vi "插入数据库.vi"(8 "时间戳":string, 9 "插入数值":string[](array[string]), 10 "table":string="多参数", 11 "database":string="database1.mdb") -> ()   [LabVIEW 2016]
uses:
  <vilib>/Utility/sysdir.llb/System Directory Type.ctl
  <vilib>/addons/database/Connection.llb/DB Tools Open Connec (String).vi
  <vilib>/addons/database/Connection.llb/Conn Execute.vi
  <vilib>/addons/database/Recordset.llb/Rec Destroy - Connection.vi
  <vilib>/addons/database/NI_Database_API.lvlib
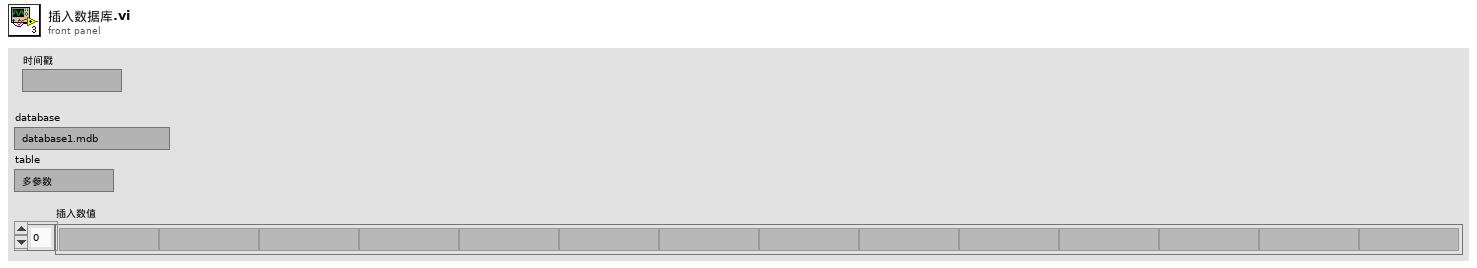
[diagram p1: front panel]
types:
  T1 = typedef "System Directory Type.ctl" = i32
  T2 = typedef "NI_Database_API.lvlib/Conn ObjectReference.ctl" = refnum<k1>
  T3 = typedef "NI_Database_API.lvlib/Rec ObjectReference.ctl" = refnum<k1>
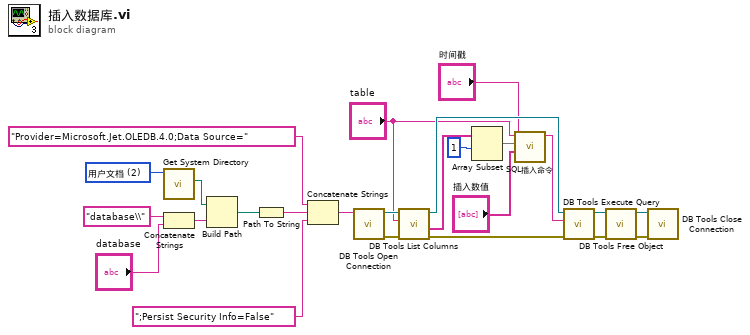
[diagram p0: block diagram]
diagram:
  w21 = T1 2 items=["用户目录"=0, "用户桌面"=1, "用户文档"=2, "用户应用程序数据"=3, "用户设置"=4, "用户临时目录"=5, "公共文档"=6, "公共应用程序数据"=7, "公共设置"=8, "公共缓存"=13, "系统核心库"=9, "系统安装库"=10, "应用程序文件"=11, "启动盘根目录"=12] ("system directory type")
  n1 = call <vilib>:"Get System Directory.vi"("system directory type"=w21) -> ("system directory"=w20:path)  [unwired: 10 in]
  n2 = Concatenate Strings("database\\" ("名称或相对路径"), "database") -> (w4:string)
  n3 = Build Path(base path=w20, name or relative path=w4) -> (appended path=w22:path)
  n4 = Path To String(path=w22) -> (string=w23:string)
  n5 = Concatenate Strings("Provider=Microsoft.Jet.OLEDB.4.0;Data Source=", w23, ";Persist Security Info=False") -> (w19:string)
  n6 = call-poly <vilib>:"DB Tools Open Connection.vi"("connection information"=w19) -> ("error out"=w17:errorcluster, "connection reference"=w18:T2)  [unwired: 7 in]
  n7 = call <vilib>:"DB Tools List Columns.vi"("error in (no error)"=w17, "table"="table", "connection reference"=w18) -> ("error out"=w10:errorcluster, "columns"=w16:string[], "connection reference out"=w11:T2)  [unwired: 1 in, 1 out]
  n8 = Array Subset(array=w16, index=1 ("索引")) -> (w14:string[])  [unwired: 1 in]
  n9 = call "SQL插入命令.vi"("时间戳"="时间戳", "插入数值"="插入数值", "段名"=w14, "table"="table") -> ("SQL插入命令"=w7:string)  [unwired: 7 in]
  n10 = call-poly <vilib>:"DB Tools Execute Query.vi"("error in (no error)"=w10, "SQL query"=w7, "connection reference"=w11) -> ("error out"=w12:errorcluster, "recordset reference"=w13:T3)  [unwired: 5 in]
  n11 = call-poly <vilib>:"DB Tools Free Object.vi"("error in (no error)"=w12, "recordset reference"=w13) -> ("error out"=w8:errorcluster, "connection reference"=w9:T2)  [unwired: 8 in]
  n12 = call <vilib>:"DB Tools Close Connection.vi"("error in (no error)"=w8, "connection reference"=w9) -> ()  [unwired: 5 in, 1 out]
